vi "Charger, Verify Unable to Reopen Session.vi"(0 "error in":errorcluster, 4 "Status Refnum":T1) -> (7 "error out":errorcluster)   [LabVIEW 2020]
uses:
  Charger_Status Refnum.ctl
  Drivers/Charger Test Set/Charger_Input Control.ctl
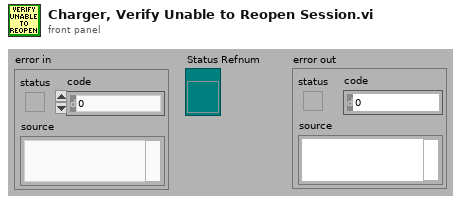
[diagram p1: front panel]
types:
  T1 = typedef "Charger_Status Refnum.ctl" = refnum<vi>
  T2 = typedef "MICS_Input Control.ctl" = cluster{"address":refnum<visa-resource-name>, "chan":u16, "ID":u32}
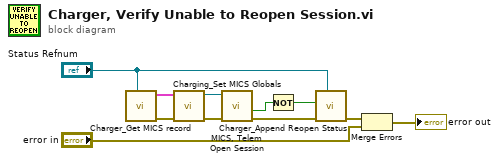
[diagram p0: block diagram]
diagram:
  n1 = call "Charger_Get MICS record.vi"("Status Refnum"="Status Refnum") -> ("error out"=w10:errorcluster, "MICS Inputs"=w9:T2)  [unwired: 4 in, 3 out]
  n2 = call "Charging_Set MICS Globals.vi"("error in"=w10, "MICS inputs"=w9) -> ("error out"=w7:errorcluster, "address"=w8:refnum<visa-resource-name>)  [unwired: 4 in]
  n3 = call "MICS, Telem Open Session.vi"("error in"=w7, "VISA resource"=w8) -> ("error out"=w6:errorcluster, "in_session"=w5:bool)  [unwired: 7 in, 1 out]
  n4 = Not(x=w5) -> (.not. x?=w4:bool)
  n5 = call "Charger_Append Reopen Status.vi"("Status Refnum"="Status Refnum", "error in"=w6, "NOT In Session"=w4) -> ("error out"=w3:errorcluster)  [unwired: 6 in]
  n6 = Merge Errors(w3, "error in") -> (→"error out":errorcluster)
